vi "ArrayRead.140620.vi"   [LabVIEW 2013]
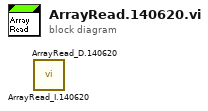
[diagram p0: block diagram]
diagram:
  n1 = call "ArrayRead_I.140620.vi"() -> ()  [unwired: 7 in, 9 out]
  n2 = call "ArrayRead_D.140620.vi"() -> ()  [unwired: 7 in, 9 out]
